vi "Mexa MAX FPGA U.vi"() -> ()   [LabVIEW 2011]
panel:
  out "Output":u8[](array[numeric])
  in  "Numeric":i16
  # "0 - measurement\n1 - start measurement\n2 - stand by"
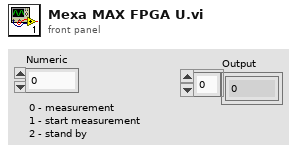
[diagram p1: front panel]
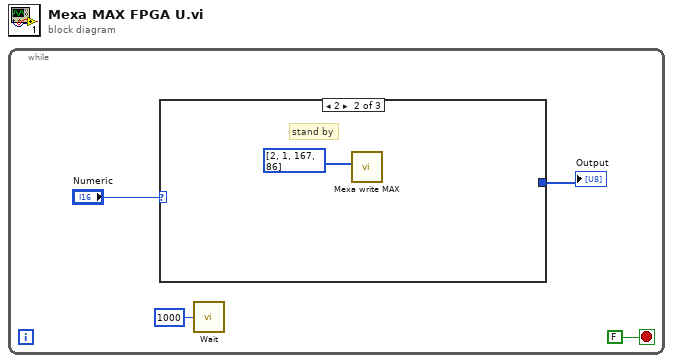
[diagram p0: block diagram]
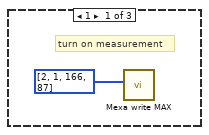
[diagram p2: hidden frame]
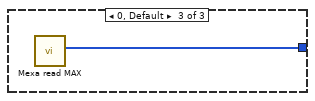
[diagram p3: hidden frame]
diagram:
  n1 = while {
    stop <- FALSE stop-if-true
    n2 = case shown="2" "Numeric" {
      tunnel: [_ _ w7] -> w3
      frame 1 {
        # "turn on measurement"
        n3 = call "Mexa write MAX.vi"("Array"=u8[] [2, 1, 166, 87]) -> ()  [unwired: 11 in]
      }
      frame 2 {
        # "stand by"
        n4 = call "Mexa write MAX.vi"("Array"=u8[] [2, 1, 167, 86]) -> ()  [unwired: 11 in]
      }
      frame 0, Default {
        n5 = call "Mexa read MAX.vi"() -> ("Output"=w7:u8[])  [unwired: 11 in]
      }
    }
    "Output" <- w3
    n6 = call "Wait"("Count(mSec)"=u32 1000) -> ()  [unwired: 1 out]
  }
